vi "Shutter Box State.vi"(8 "error in (no error)":errorcluster) -> ()   [LabVIEW 2016]
uses:
  Controls/Operational Modes.ctl
  Controls/Shutters.ctl
  Controls/Shutter Data.ctl
  Controls/Shutter States.ctl
  Controls/Shutter Box State.ctl
panel:
  out "error out":errorcluster
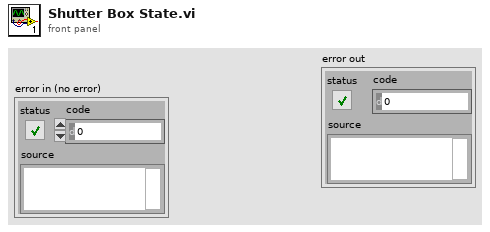
[diagram p1: front panel]
types:
  T1 = typedef "Operational Modes.ctl" = enum16{"Sci", "Sci-LFC", "Solar", "Solar-LFC", "LFC", "LFC-Sim", "LFC-Both", "ThAr", "ThAr-LFC", "Flat", "ExtFlat", "ExtFlat-Sim", "ExtFlat-Both", "Qtz", "ExtQtz", "ExtQtz-Sim", "ExtQtz-Both", "Dark", "Manual", "Off"}
  T2 = typedef "Shutters.ctl" = cluster{"Science":T3, "LFCSim":T3, "ExtendFlat":T3, "SimFlat":T3, "Solar":T3}
  T3 = typedef "Shutter Data.ctl" = cluster{"Status":bool, "State":T4, "Time Stamps":cluster{"Open":timestamp, "Close":timestamp}, "Exposure Time":dbl}
  T4 = typedef "Shutter States.ctl" = enum16{"Open", "Close", "Wait", "Off", "Arm", "Idle"}
  T5 = typedef "Shutter Box State.ctl" = enum16{"Idle", "Armed", "Integrating"}
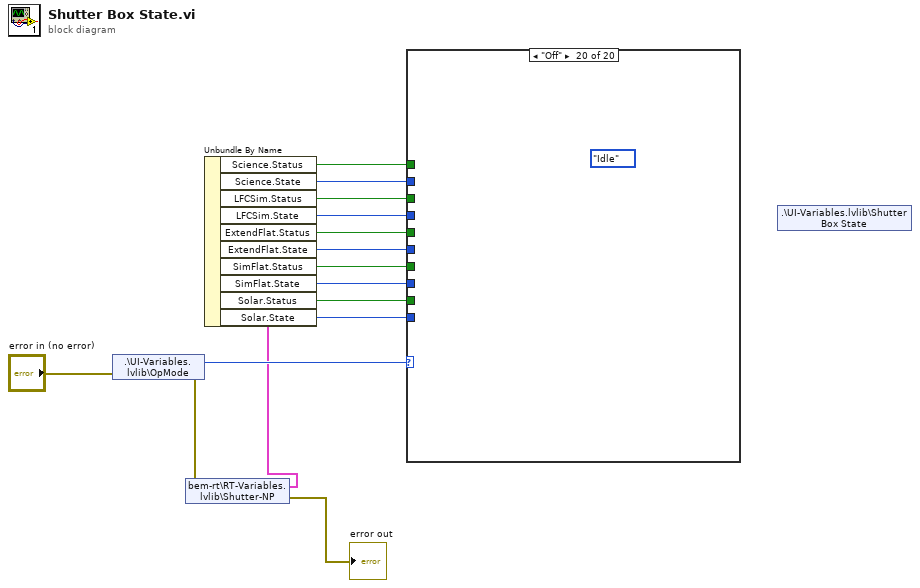
[diagram p0: block diagram]
diagram:
  n1 = shared-variable ".\\UI-Variables.lvlib\\OpMode"(error in="error in (no error)") -> (w12:T1, error out=w15:errorcluster)
  n2 = shared-variable "bem-rt\\RT-Variables.lvlib\\Shutter-NP"(error in=w15) -> (w11:T2, error out=→"error out":errorcluster)
  n3 = Unbundle By Name(w11) -> ("Science.Status"=w10:bool, "Science.State"=w9:T4, "LFCSim.Status"=w8:bool, "LFCSim.State"=w7:T4, "ExtendFlat.Status"=w6:bool, "ExtendFlat.State"=w5:T4, "SimFlat.Status"=w4:bool, "SimFlat.State"=w3:T4, "Solar.Status"=w2:bool, "Solar.State"=w1:T4)
  n4 = case shown="\"Off\"" w12 {
    tunnel: w10 -> [_ _ _ _ _ _ _ _ _ _ _ _ _ _ _ _ _ _ _ _]
    tunnel: w9 -> [_ _ _ _ _ _ _ _ _ _ _ _ _ _ _ _ _ _ _ _]
    tunnel: w8 -> [_ _ _ _ _ _ _ _ _ _ _ _ _ _ _ _ _ _ _ _]
    tunnel: w7 -> [_ _ _ _ _ _ _ _ _ _ _ _ _ _ _ _ _ _ _ _]
    tunnel: w6 -> [_ _ _ _ _ _ _ _ _ _ _ _ _ _ _ _ _ _ _ _]
    tunnel: w5 -> [_ _ _ _ _ _ _ _ _ _ _ _ _ _ _ _ _ _ _ _]
    tunnel: w4 -> [_ _ _ _ _ _ _ _ _ _ _ _ _ _ _ _ _ _ _ _]
    tunnel: w3 -> [_ _ _ _ _ _ _ _ _ _ _ _ _ _ _ _ _ _ _ _]
    tunnel: w2 -> [_ _ _ _ _ _ _ _ _ _ _ _ _ _ _ _ _ _ _ _]
    tunnel: w1 -> [_ _ _ _ _ _ _ _ _ _ _ _ _ _ _ _ _ _ _ _]
    frame "Sci", Default {
    }
    frame "Sci-LFC" {
    }
    frame "Solar" {
    }
    frame "Solar-LFC" {
    }
    frame "LFC" {
    }
    frame "LFC-Sim" {
    }
    frame "LFC-Both" {
    }
    frame "ThAr" {
    }
    frame "ThAr-LFC" {
    }
    frame "Flat" {
    }
    frame "ExtFlat" {
    }
    frame "ExtFlat-Sim" {
    }
    frame "ExtFlat-Both" {
    }
    frame "Qtz" {
    }
    frame "ExtQtz" {
    }
    frame "ExtQtz-Sim" {
    }
    frame "ExtQtz-Both" {
    }
    frame "Dark" {
    }
    frame "Manual" {
    }
    frame "Off" {
      (unwired) Shutter_Box_State."Idle" ("Shutter box state")
    }
  }
  n5 = shared-variable ".\\UI-Variables.lvlib\\Shutter Box State"() -> ()  [unwired: 2 in, 1 out]
